vi "Monitor Data Changed.vi"(8 "error in (no error)":errorcluster, 9 "Changed Actor's Q":refnum<class "Message Enqueuer.lvclass">, 10 "Monitor Data":refnum<class "Monitor Data.lvclass">, 11 "Debug Monitor New in":refnum<class "Debug Monitor.lvclass">) -> (0 "error out":errorcluster, 3 "Debug Monitor New out":refnum<class "Debug Monitor.lvclass">)   [LabVIEW 2017, in "Debug Monitor.lvclass"]
doc: "Called any time the monitor data is changed. Use the \"Changed Actor's Q\" to determine what actor has changed.\n\nCopyright: MGI 2016\nAuthor: Derek Trepanier"
uses:
  Debug Monitor.lvclass
  Source/Monitor Data/Monitor Data.lvclass
  <vilib>/ActorFramework/Message Enqueuer/Message Enqueuer.lvclass
  Debug Monitor.lvclass/Debug Monitor.ctl
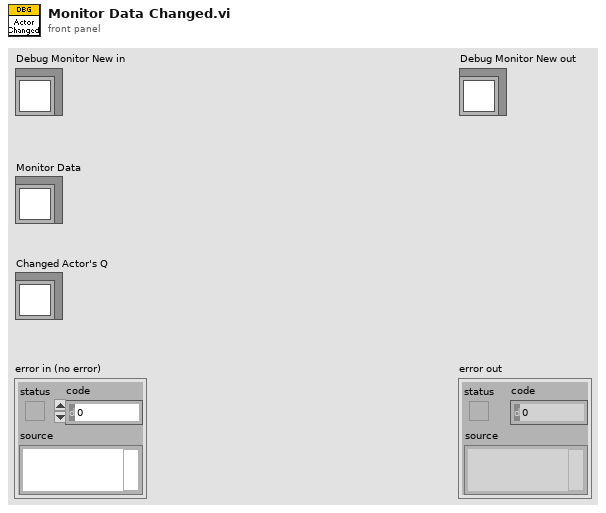
[diagram p1: front panel]
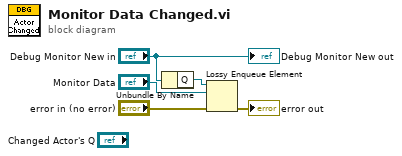
[diagram p0: block diagram]
diagram:
  n1 = Unbundle By Name("Debug Monitor New in") -> ("Q"=w4:refnum<queue>)
  n2 = Lossy Enqueue Element(queue=w4, element="Monitor Data", error in (no error)="error in (no error)") -> (error out=→"error out":errorcluster)  [unwired: 3 out]
  "Debug Monitor New out" <- "Debug Monitor New in"
